vi "Experiment_opticalfiber_Bend.vi"() -> ()   [LabVIEW 2009]
uses:
  <vilib>/imath/engines/lvmath2/RunTimeEngine/ErrorHandling/NIMS_Finalize Error.vi
  <vilib>/imath/engines/lvmath2/RunTimeEngine/Parser/MC_Version.vi
  <vilib>/imath/engines/lvmath/Functions/Error Handling/error.ctl
  <vilib>/imath/engines/lvmath2/RunTimeEngine/RangeToken/NIMS_Range.vi
  <instcachedir>/0/NIMS_Range_6D647EC16A744C98B5DE1D649A2D648D.lvgen/NIMS_Range_6D647EC16A744C98B5DE1D649A2D648D_001.vi
  <vilib>/imath/engines/lvmath2/RunTimeEngine/VariableToken/NIMS_VariableToken_CondDefined.vi
  <instcachedir>/0/NIMS_VariableToken_CondDefined_5641E79000FB4D628475532441475385.lvgen/NIMS_VariableToken_CondDefined_5641E79000FB4D628475532441475385_002.vi
  <vilib>/imath/engines/lvmath/Functions/Error Handling/MC_Mask_Errors.vi
  <vilib>/imathl/engines/lvmath/Functions/Error Handling/Create Error.vi
  <vilib>/imath/engines/lvmath2/RunTimeEngine/ReplaceToken/NIMS_Replace - V(S)=S.vi
  <instcachedir>/0/NIMS_Replace - V(S)=S_670A9E0533664C1D848C8E58B3321B6A.lvgen/NIMS_Replace - V(S)=S_670A9E0533664C1D848C8E58B3321B6A_000.vi
  <vilib>/imath/engines/lvmath2/RunTimeEngine/ReplaceToken/NIMS_Replace - Size Check _(_)=S.vi
  <instcachedir>/0/NIMS_Replace - Size Check _(_)=S_8596181D73404097BAB9CBB006194BB0.lvgen/NIMS_Replace - Size Check _(_)=S_8596181D73404097BAB9CBB006194BB0_001.vi
  <vilib>/imath/engines/lvmath2/RunTimeEngine/ReplaceToken/NIMS_Replace - Check Linear.vi
  <instcachedir>/0/NIMS_Replace - Check Linear_9243CBB174894FF6977027453DA6955E.lvgen/NIMS_Replace - Check Linear_9243CBB174894FF6977027453DA6955E_001.vi
  <vilib>/imath/engines/lvmath2/RunTimeEngine/VariableToken/NIMS_VariableToken_CondDefinedDefinedByReplace.vi
  <instcachedir>/0/NIMS_VariableToken_CondDefinedDefinedByReplace_D162CFFC24174562A9FEA619A91E1A56.lvgen/NIMS_VariableToken_CondDefinedDefinedByReplace_D162CFFC24174562A9FEA619A91E1A56_001.vi
  <instcachedir>/0/NIMS_Replace - V(S)=S_670A9E0533664C1D848C8E58B3321B6A.lvgen/NIMS_Replace - V(S)=S_670A9E0533664C1D848C8E58B3321B6A_001.vi
  <instcachedir>/0/NIMS_Replace - Size Check _(_)=S_8596181D73404097BAB9CBB006194BB0.lvgen/NIMS_Replace - Size Check _(_)=S_8596181D73404097BAB9CBB006194BB0_002.vi
  <instcachedir>/0/NIMS_Replace - Check Linear_9243CBB174894FF6977027453DA6955E.lvgen/NIMS_Replace - Check Linear_9243CBB174894FF6977027453DA6955E_002.vi
  <instcachedir>/0/NIMS_VariableToken_CondDefinedDefinedByReplace_D162CFFC24174562A9FEA619A91E1A56.lvgen/NIMS_VariableToken_CondDefinedDefinedByReplace_D162CFFC24174562A9FEA619A91E1A56_002.vi
  <vilib>/imath/engines/lvmath2/RunTimeEngine/CommandStatement/MC_CommandStatement_break.vi
  <vilib>/imath/engines/lvmath2/RunTimeEngine/Managers/WorkSpace/UID Generator.vi
  <vilib>/imath/engines/lvmath2/RunTimeEngine/Managers/SymbolTable/Clear UID.vi
  <instcachedir>/0/NIMS_VariableToken_CondDefined_5641E79000FB4D628475532441475385.lvgen/NIMS_VariableToken_CondDefined_5641E79000FB4D628475532441475385_003.vi
  <vilib>/imath/engines/lvmath/Functions/Error Handling/MergeErrorsWrapper.vi
  <instcachedir>/0/NIMS_Replace - V(S)=S_670A9E0533664C1D848C8E58B3321B6A.lvgen/NIMS_Replace - V(S)=S_670A9E0533664C1D848C8E58B3321B6A_002.vi
  <instcachedir>/0/NIMS_Replace - Size Check _(_)=S_8596181D73404097BAB9CBB006194BB0.lvgen/NIMS_Replace - Size Check _(_)=S_8596181D73404097BAB9CBB006194BB0_003.vi
  <vilib>/imath/engines/lvmath2/RunTimeEngine/ArithmeticOperatorToken/NIMS_ArithmeticOperator_power(S).vi
  <instcachedir>/0/NIMS_ArithmeticOperator_power(S)_A502679C095F4520BDC53E297C98A9BD.lvgen/NIMS_ArithmeticOperator_power(S)_A502679C095F4520BDC53E297C98A9BD_000.vi
  <instcachedir>/0/NIMS_Replace - Check Linear_9243CBB174894FF6977027453DA6955E.lvgen/NIMS_Replace - Check Linear_9243CBB174894FF6977027453DA6955E_003.vi
  <instcachedir>/0/NIMS_VariableToken_CondDefinedDefinedByReplace_D162CFFC24174562A9FEA619A91E1A56.lvgen/NIMS_VariableToken_CondDefinedDefinedByReplace_D162CFFC24174562A9FEA619A91E1A56_003.vi
  <vilib>/imath/engines/lvmath2/RunTimeEngine/LocalVariableDefStatement/MC_LocalVariableDefStatement_Display.vi
  <vilib>/imath/engines/lvmath2/RunTimeEngine/RunTimeType/NIMS_RunTimeType_From StrictType (excl LVString).vi
  <vilib>/imath/engines/lvmath2/RunTimeEngine/VariableToken/Read/NIMS_Get Elements - RV(_) - Check.vi
  <instcachedir>/0/NIMS_Get Elements - RV(_) - Check_60F12861D0564803969A5D0D0D1716CD.lvgen/NIMS_Get Elements - RV(_) - Check_60F12861D0564803969A5D0D0D1716CD_002.vi
  <instcachedir>/0/NIMS_ArithmeticOperator_power(S)_A502679C095F4520BDC53E297C98A9BD.lvgen/NIMS_ArithmeticOperator_power(S)_A502679C095F4520BDC53E297C98A9BD_001.vi
  <instcachedir>/0/NIMS_ArithmeticOperator_power(S)_A502679C095F4520BDC53E297C98A9BD.lvgen/NIMS_ArithmeticOperator_power(S)_A502679C095F4520BDC53E297C98A9BD_003.vi
  <vilib>/imath/engines/lvmath2/RunTimeEngine/Managers/SymbolTable/NIMS_WorkSpace.lvlib
panel:
  in  "HELP FOR FIBER LENGTH":bool
  out "error out":errorcluster
  out "error out":errorcluster
  in  "?":bool
  in  "?":enum32{"NUMBER OF TURNS OF FIBER"}(tab)
  in  "?":T1(radio)
  in  "?":enum32{"OSCILLOSCOPE"}(tab)
  out "?":dbl[](graph)
  in  "HELP FOR CRO":bool
  in  "?":enum32{"STEP FUNCTION GENRATOR"}(tab)
  out "?":dbl[](graph)
  in  "HELP FOR SOURCE":bool
  out "error out":errorcluster
  # "Function generator"
  # "Oscilloscope"
  # "ON"
  # "OFF"
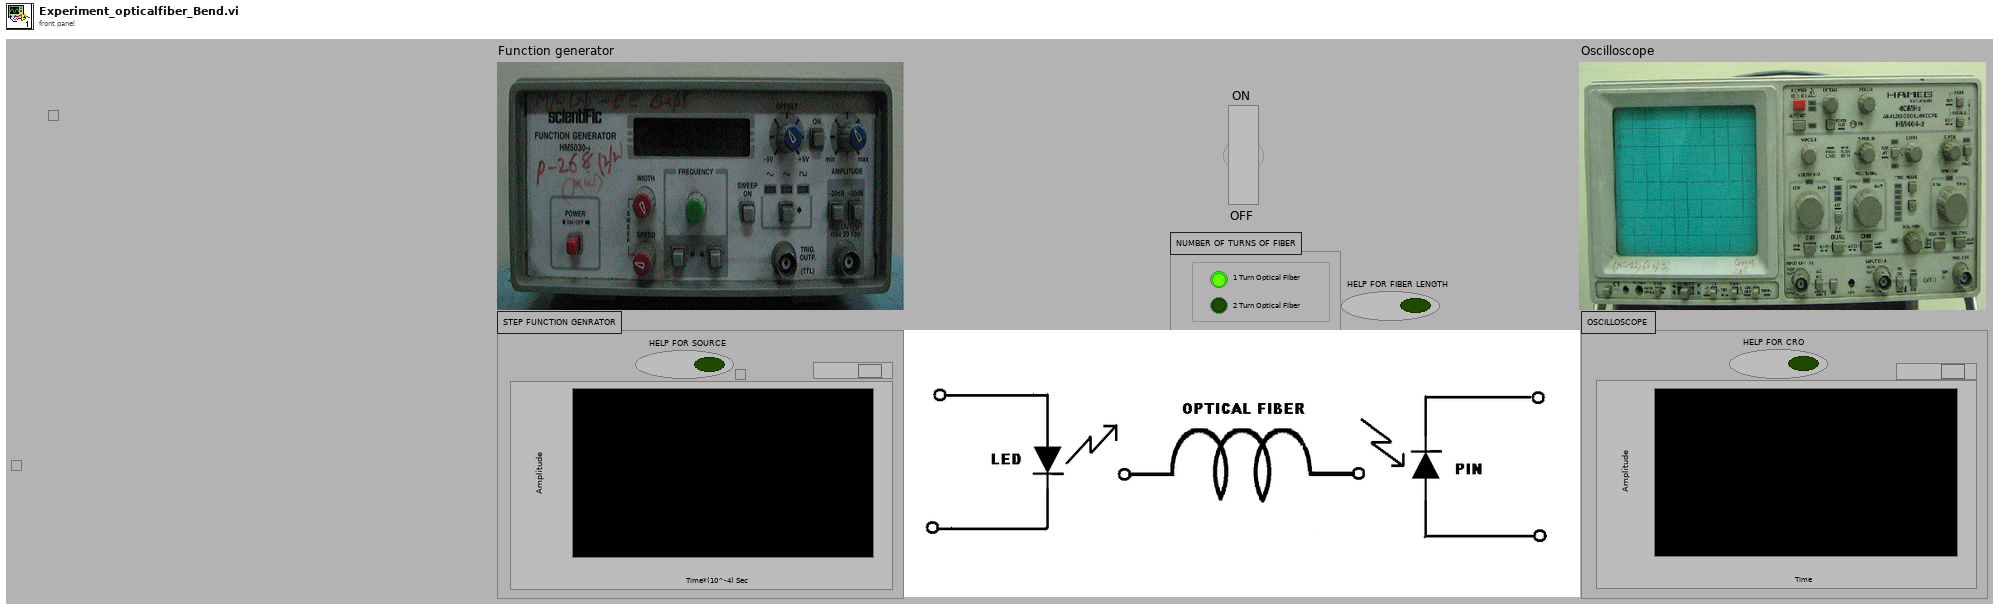
[diagram p1: front panel]
types:
  T1 = enum32{"1 Turn Optical Fiber", " 2 Turn Optical Fiber"}
  T2 = typedef "error.ctl" = enum16{"No Error", "Problem", "Unused002", "Incorrect number of parameters", "Function not defined for non-numeric types", "Unused005", "Function only defined for character arrays", "Function not defined for boolean, character, or single precision", "Function not defined for complex types", "Not a valid operation", "Inputs must be scalar", "Input matrices are not the same size", "Unused012", "Input matrices must be nonnegative integers of the same type", "Arguments must be non-negative integers less than bitmax", "Number to complement must be less than 2^N", "Bit to get is outside range", "Bit to set is outside range", "Input must be real type ", "At least one parameter must be scalar", "Unused020", "Function not defined for\nhigher dimensional matrices.", "Invalid attributes", "Wrong Type of Input Arguments", "Wrong Argument Option", "Unused025", "Indices must be real positive integers", "Unused027", "Number of elements must be the same for indices and values", "Unused029", "Cannot resize a 2D matrix with a linear index", "Unknown variable or symbol", "Indices out of range", "Empty matrix deletion can not be used with two indices", "Number of rows and columns must be the same for indices and values.", "Complex cannot be converted to Boolean", "Char cannot be converted to Boolean", "int64 cannot be converted to Boolean", "uint64 cannot be converted to Boolean", "Unused039", "Unused040", "All rows must have the same number of columns", "Incompatible types", "Invalid matrix dimensions", "Dimension must be 1 or 2", "Base must be an integer between 2 and 36", "Invalid input", "Square matrix required", "Function 'timerstart' must be called before 'timerstop'", "Arguments must be positive real", "Step must not be zero", "Wrong number of input arguments", "Wrong number of output arguments", "Unused053", "Input scalar must be >= 0", "Input scalar must be positive", "Input scalar must not be 0", "Input scalar must be in range [0,1]", "Unused058", "Input must be a vector", "Unused060", "Empty vector error", "All elements must be in domain [-1,1]", "All real elements of input vector must be >= 0", "All elements of input vector must be positive", "Values of input vectors are not compatible", "Unused066", "Input vector must be an increasing vector", "Unused068", "Unused069", "Lenths of two input vectors are not compatible", "Unused071", "Empty matrix error", "Unused073", "Unused074", "Unused075", "Unused076", "Unused077", "Size of input matrix is incompatible with input size", "Invalid format specifier", "Unused080", "Unused081", "Unused082", "Unused083", "Unused084", "Unused085", "RunTime: MathScript could not be compiled", "Unknown function", "Only scalars and strings supported", "Unused089", "Unused090", "Range is too large", "End used without variable", "Function not available (RTE)", "Custom user error", "Arguments must be integers less than bitmax", "Shared library not found", "Header file not found", "Shared library already loaded", "Shared library not loaded", "Shared library function not found", "Shared library string return problem", "Problem calling shared library function", "Problem loading shared library from OS", "Problem parsing shared library header file", "Shared library incompatible types", "Shared library unsupported return type", "Shared library function not exported", "Shared library unsupported input type", "Problem unloading shared library from OS", "Function only available from UI", "Invalid function specified in argument", "An internal error has occurred", "Invalid object", "Invalid property", "Read-only property", "A break command has occurred", "A continue command has occurred", "A return command has occurred", "ode: times parameter invalid", "Unused120", "Function not found in file", "Reserved keyword cannot be defined as variable", "Reserved keyword cannot be defined as a function or script", "Arguments must be string literals", "Function not supported on this platform", "All columns must have the same number of rows", "Function ignored in RTE warning", "Cannot use : as a parameter that is not a variable", "Output can't be coerced to requested type", "Function not supported on current target", "Variable dependent on an unwired function input", "Unused132", "Unused133", "Unused134", "Unused135", "Unused136", "Unused137", "Unused138", "Unused139", "Unused140", "Unused141", "Unused142", "Unused143", "Unused144", "Unused145", "Unused146", "MathScript parser DLL missing", "MathScript requires LabVIEW Full", "MathScript license is invalid or missing"}
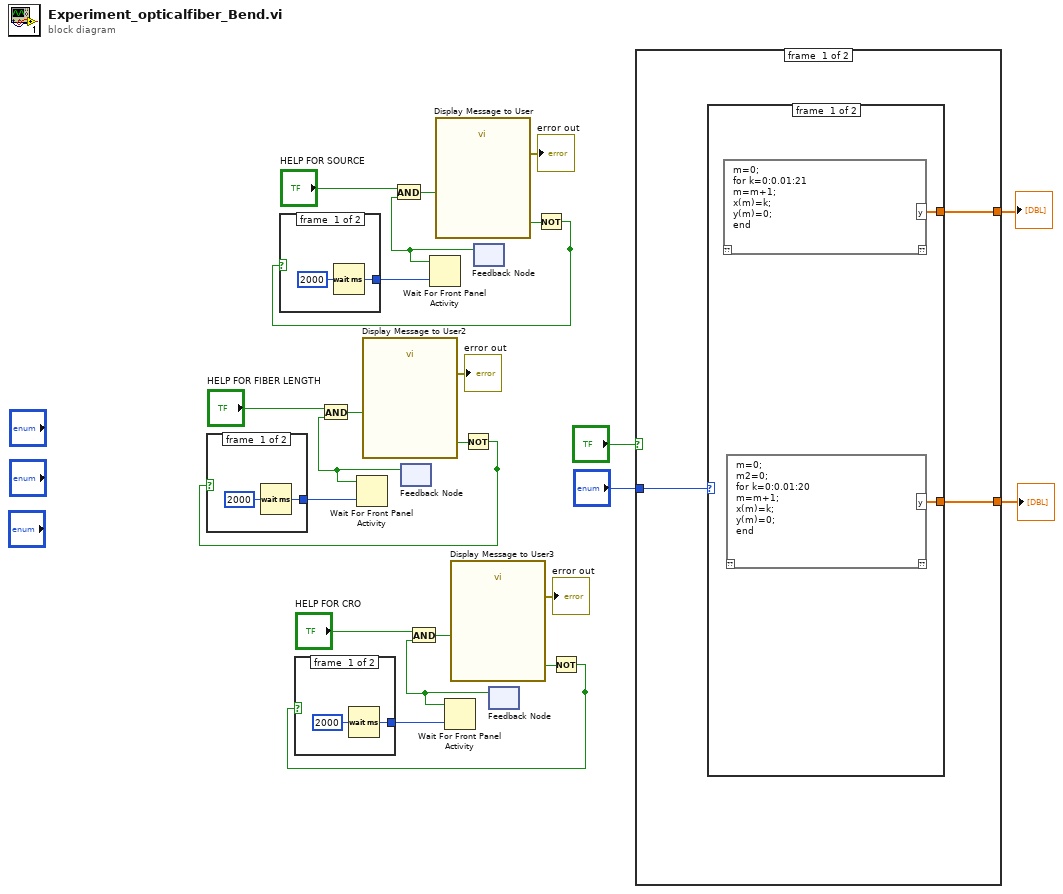
[diagram p0: block diagram]
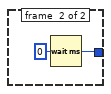
[diagram p2: hidden frame]
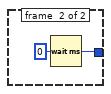
[diagram p3: hidden frame]
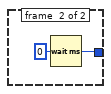
[diagram p4: hidden frame]
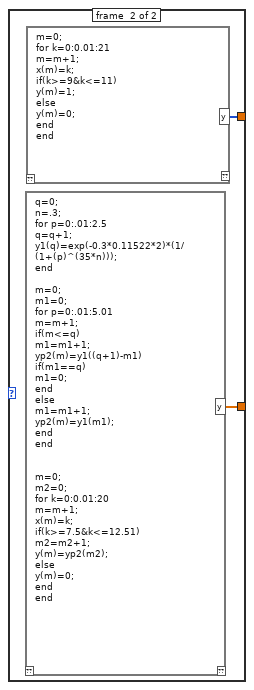
[diagram p5: hidden frame]
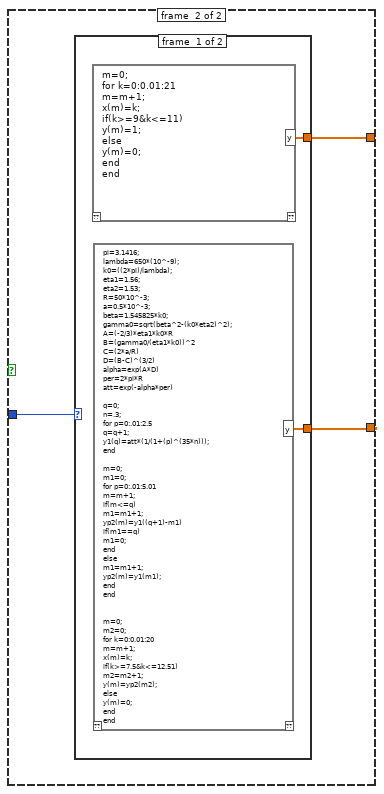
[diagram p6: hidden frame]
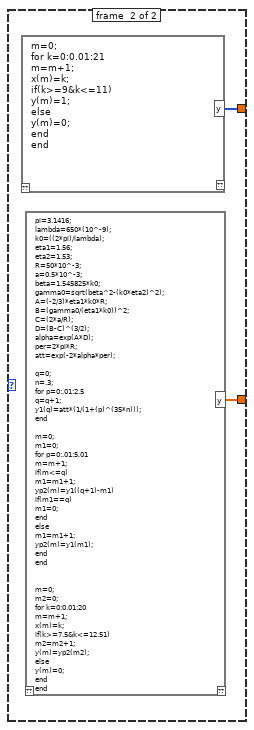
[diagram p7: hidden frame]
diagram:
  n1 = feedback #1() -> (w13:bool)  [unwired: 1 in]
  n2 = And(x="HELP FOR FIBER LENGTH", y=w13) -> (x .and. y?=w14:bool)
  n3 = call "Display Message to User2"("Enable"=w14) -> ("error out"=→"error out":errorcluster, "CLOSE"=w12:bool)  [unwired: 2 in, 7 out]
  n4 = Not(x=w12) -> (.not. x?=w10:bool)
  n5 = case shown="False" w10 {
    tunnel: [w26 w28] -> w9
    frame #0 {
      n6 = Wait (ms)(milliseconds to wait=u32 2000) -> (millisecond timer value=w26:u32)
    }
    frame #1 {
      n7 = Wait (ms)(milliseconds to wait=u32 0) -> (millisecond timer value=w28:u32)
    }
  }
  n8 = Wait For Front Panel Activity(1:w9, 3:w13) -> ()  [unwired: 1 in, 1 out]
  n9 = feedback #2() -> (w20:bool)  [unwired: 1 in]
  n10 = And(x="HELP FOR SOURCE", y=w20) -> (x .and. y?=w21:bool)
  n11 = call "Display Message to User"("Enable"=w21) -> ("error out"=→"error out":errorcluster, "CLOSE"=w19:bool)  [unwired: 2 in, 7 out]
  n12 = feedback #3() -> (w6:bool)  [unwired: 1 in]
  n13 = And(x="HELP FOR CRO", y=w6) -> (x .and. y?=w7:bool)
  n14 = call "Display Message to User3"("Enable"=w7) -> ("error out"=→"error out":errorcluster, "CLOSE"=w5:bool)  [unwired: 2 in, 7 out]
  n15 = Not(x=w19) -> (.not. x?=w17:bool)
  n16 = case shown="False" w17 {
    tunnel: [w30 w32] -> w16
    frame #0 {
      n17 = Wait (ms)(milliseconds to wait=u32 2000) -> (millisecond timer value=w30:u32)
    }
    frame #1 {
      n18 = Wait (ms)(milliseconds to wait=u32 0) -> (millisecond timer value=w32:u32)
    }
  }
  n19 = Wait For Front Panel Activity(1:w16, 3:w20) -> ()  [unwired: 1 in, 1 out]
  n20 = Not(x=w5) -> (.not. x?=w3:bool)
  n21 = case shown="False" w3 {
    tunnel: [w34 w36] -> w2
    frame #0 {
      n22 = Wait (ms)(milliseconds to wait=u32 2000) -> (millisecond timer value=w34:u32)
    }
    frame #1 {
      n23 = Wait (ms)(milliseconds to wait=u32 0) -> (millisecond timer value=w36:u32)
    }
  }
  n24 = Wait For Front Panel Activity(1:w2, 3:w6) -> ()  [unwired: 1 in, 1 out]
  n25 = case shown="False" "?" {
    tunnel: [w40 w958] -> w24
    tunnel: [w39 w957] -> w23
    tunnel: "?" -> [w38 w956]
    frame #0 {
      n26 = case shown="\"1 Turn Optical Fiber\", Default" w38 {
        tunnel: [w42 w298] -> w39
        tunnel: [w41 w297] -> w40
        frame #0 {
          n27 = mathscript code="m=0;\nfor k=0:0.01:21\nm=m+1;\nx(m)=k;\ny(m)=0;\nend"() -> ("y"=w41:dbl[])  [unwired: 2 out]
          n28 = mathscript code="m=0;\nm2=0;\nfor k=0:0.01:20\nm=m+1;\nx(m)=k;\ny(m)=0;\nend"() -> ("y"=w42:dbl[])  [unwired: 2 out]
        }
        frame #1 {
          n29 = mathscript code="q=0;\nn=.3;\nfor p=0:.01:2.5\nq=q+1;\ny1(q)=exp(-0.3*0.11522*2)*(1/(1+(p)^(35*n)));\nend\n\nm=0;\nm1=0;\nfor p=0:.01:5.01\nm=m+1;\nif(m<=q)\nm1=m1+1;\nyp2(m)=y1((q+1)-m1)\nif(m1==q)\nm1=0;\nend\nelse\nm1=m1+1;\nyp2(m)=y1(m1);\nend\nend\n\n\nm=0;\nm2=0;\nfor k=0:0.01:20\nm=m+1;\nx(m)=k;\nif(k>=7.5&k<=12.51)\nm2=m2+1;\ny(m)=yp2(m2);\nelse\ny(m)=0;\nend\nend"() -> ("y"=w298:dbl[])  [unwired: 2 out]
          n30 = mathscript code="m=0;\nfor k=0:0.01:21\nm=m+1;\nx(m)=k;\nif(k>=9&k<=11)\ny(m)=1;\nelse\ny(m)=0;\nend\nend"() -> ("y"=w297:i32[])  [unwired: 2 out]
        }
      }
    }
    frame #1 {
      n31 = case shown="\"1 Turn Optical Fiber\", Default" w956 {
        tunnel: [w960 w1822] -> w957
        tunnel: [w959 w1821] -> w958
        frame #0 {
          n32 = mathscript code="m=0;\nfor k=0:0.01:21\nm=m+1;\nx(m)=k;\nif(k>=9&k<=11)\ny(m)=1;\nelse\ny(m)=0;\nend\nend"() -> ("y"=w959:dbl[])  [unwired: 2 out]
          n33 = mathscript code="pi=3.1416;\nlambda=650*(10^-9);\nk0=((2*pi)/lambda);\neta1=1.56;\neta2=1.53;\nR=50*10^-3;\na=0.5*10^-3;\nbeta=1.545825*k0;\ngamma0=sqrt(beta^2-(k0*eta2)^2);\nA=(-2/3)*eta1*k0*R\nB=(gamma0/(eta1*k0))^2\nC=(2*a/R)\nD=(B-C)^(3/2)\nalpha=exp(A*D)\nper=2*pi*R\natt=exp(-alpha*per)\n\nq=0;\nn=.3;\nfor p=0:.01:2.5\nq=q+1;\ny1(q)=att*(1/(1+(p)^(35*n)));\nend\n\nm=0;\nm1=0;\nfor p=0:.01:5.01\nm=m+1;\nif(m<=q)\nm1=m1+1;\nyp2(m)=y1((q+1)-m1)\nif(m1==q)\nm1=0;\nend\nelse\nm1=m1+1;\nyp2(m)=y1(m1);\nend\nend\n\n\nm=0;\nm2=0;\nfor k=0:0.01:20\nm=m+1;\nx(m)=k;\nif(k>=7.5&k<=12.51)\nm2=m2+1;\ny(m)=yp2(m2);\nelse\ny(m)=0;\nend\nend"() -> ("y"=w960:dbl[])  [unwired: 2 out]
        }
        frame #1 {
          n34 = mathscript code="m=0;\nfor k=0:0.01:21\nm=m+1;\nx(m)=k;\nif(k>=9&k<=11)\ny(m)=1;\nelse\ny(m)=0;\nend\nend"() -> ("y"=w1821:i32[])  [unwired: 2 out]
          n35 = mathscript code="pi=3.1416;\nlambda=650*(10^-9);\nk0=((2*pi)/lambda);\neta1=1.56;\neta2=1.53;\nR=50*10^-3;\na=0.5*10^-3;\nbeta=1.545825*k0;\ngamma0=sqrt(beta^2-(k0*eta2)^2);\nA=(-2/3)*eta1*k0*R;\nB=(gamma0/(eta1*k0))^2;\nC=(2*a/R);\nD=(B-C)^(3/2);\nalpha=exp(A*D);\nper=2*pi*R;\natt=exp(-2*alpha*per);\n\nq=0;\nn=.3;\nfor p=0:.01:2.5\nq=q+1;\ny1(q)=att*(1/(1+(p)^(35*n)));\nend\n\nm=0;\nm1=0;\nfor p=0:.01:5.01\nm=m+1;\nif(m<=q)\nm1=m1+1;\nyp2(m)=y1((q+1)-m1)\nif(m1==q)\nm1=0;\nend\nelse\nm1=m1+1;\nyp2(m)=y1(m1);\nend\nend\n\n\nm=0;\nm2=0;\nfor k=0:0.01:20\nm=m+1;\nx(m)=k;\nif(k>=7.5&k<=12.51)\nm2=m2+1;\ny(m)=yp2(m2);\nelse\ny(m)=0;\nend\nend"() -> ("y"=w1822:dbl[])  [unwired: 2 out]
        }
      }
    }
  }
  "?" <- w24
  "?" <- w23
